vi "Write Sum.vi"(0 "TwinCAT ADS in":refnum<class "TwinCAT ADS.lvclass">, 5 ".NET Type Stream":refnum<k24>[](array[refnum]), 7 ".NET Object Stream":refnum<k24>[](array[refnum]), 9 "Handles":u32[](array[numeric]), 11 "error in (no error)":errorcluster) -> (4 "TwinCAT ADS out":refnum<class "TwinCAT ADS.lvclass">, 10 "Handles":u32[](array[numeric]), 15 "error out":errorcluster)   [LabVIEW 2018, in "TwinCAT ADS.lvclass"]
uses:
  TwinCAT ADS.lvclass
  TwinCAT.Ads
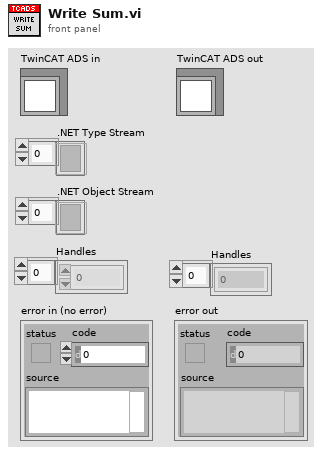
[diagram p1: front panel]
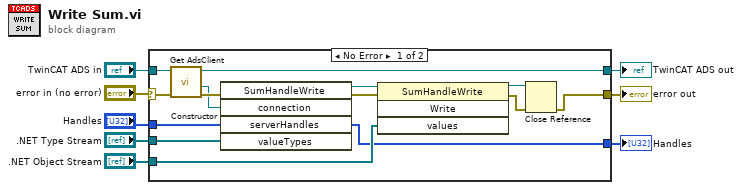
[diagram p0: block diagram]
diagram:
  n1 = case shown="No Error" "error in (no error)" {
    selector: "error in (no error)" -> [w22 w24]
    tunnel: [w20 w24] -> w7
    tunnel: [w21 w23] -> w5
    tunnel: "TwinCAT ADS in" -> [w9 w23]
    tunnel: "Handles" -> [w13 _]
    tunnel: ".NET Type Stream" -> [w12 _]
    tunnel: ".NET Object Stream" -> [w11 _]
    tunnel: [w10 _] -> w1
    frame No Error {
      n2 = call-dynamic "Get AdsClient.vi"("error in (no error)"=w22, "TwinCAT ADS in"=w9) -> ("error out"=w19:errorcluster, ".NET TcAdsClient refnum"=w14:refnum<k24>, "TwinCAT ADS out"=w21:refnum<class "TwinCAT ADS.lvclass">)  [unwired: 7 in]
      n3 = constructor class="SumHandleWrite"(error in=w19, "connection"=w14, "serverHandles"=w13, "valueTypes"=w12) -> (reference out=w17:refnum<k24>, error out=w18:errorcluster, "serverHandles"=w10:u32[])  [unwired: 2 in, 3 out]
      n4 = invoke class="SumHandleWrite" method="Write"(reference=w17, error in=w18, "values"=w11) -> (reference out=w15:refnum<k24>, error out=w16:errorcluster)  [unwired: 1 in, 2 out]
      n5 = Close Reference(reference=w15, error in (no error)=w16) -> (error out=w20:errorcluster)
    }
    frame Error {
    }
  }
  "error out" <- w7
  "TwinCAT ADS out" <- w5
  "Handles" <- w1
